vi "Write Second Level VR.vi"(5 "Tag":string, 7 "Section":string, 8 "error in (no error)":errorcluster, 10 "Value":string, 11 "Variant Repository In":variant) -> (0 "error out":errorcluster, 3 "Variant Repository Out":variant)   [LabVIEW 2017, in "Front Panel Publisher.lvlib"]
uses:
  Front Panel Publisher.lvlib
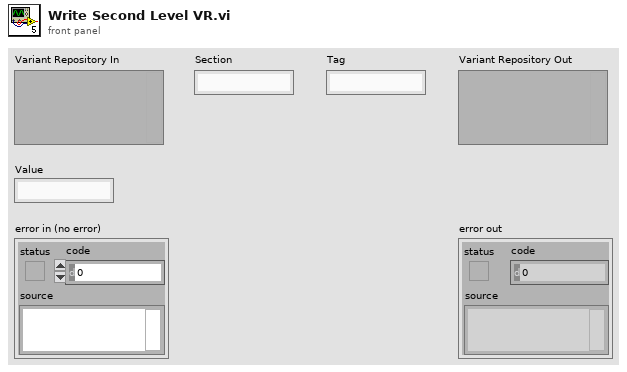
[diagram p1: front panel]
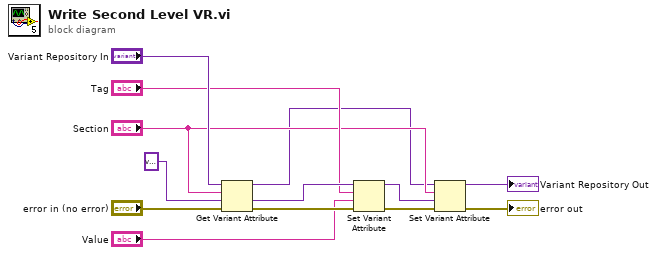
[diagram p0: block diagram]
diagram:
  n1 = Get Variant Attribute(Variant="Variant Repository In", name="Section", default value (empty Variant)=variant, error in="error in (no error)") -> (duplicate Variant=w3:variant, value=w11:variant, error out=w9:errorcluster)  [unwired: 1 out]
  n2 = Set Variant Attribute(Variant=w11, name="Tag", value="Value", error in=w9) -> (Variant out=w5:variant, error out=w7:errorcluster)  [unwired: 1 out]
  n3 = Set Variant Attribute(Variant=w3, name="Section", value=w5, error in=w7) -> (Variant out=→"Variant Repository Out":variant, error out=→"error out":errorcluster)  [unwired: 1 out]
